vi "Item.vi"(8 "error in (no error)":errorcluster, 10 "Key":string, 11 "VariantAttribute in":refnum<class "MapImp.lvclass">) -> (0 "error out":errorcluster, 1 "Value":refnum<class>, 3 "VariantAttribute out":refnum<class "MapImp.lvclass">)   [LabVIEW 2013, in "LapDog.Collections.v1.Maps.lvlib" / "MapImp.lvclass"]
doc: "Returns a copy of the value associated with the given key.\n\nIf the key does not exist, error 510203 is returned."
uses:
  MapImp.lvclass
  MapImp.lvclass/MapImp.ctl
  LapDog.Collections.Common/LapDog.Collections.v1.Common.lvlib
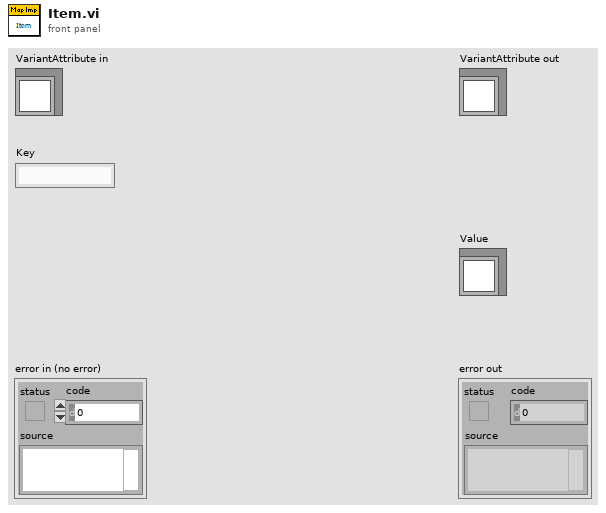
[diagram p1: front panel]
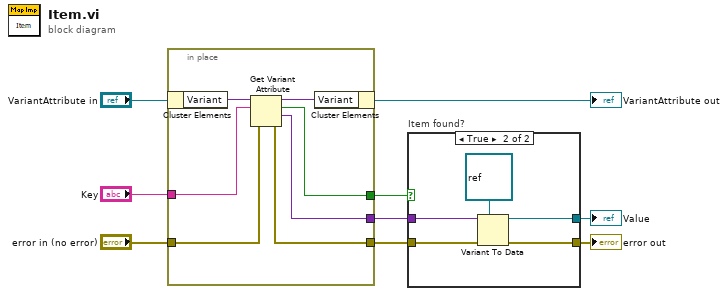
[diagram p0: block diagram]
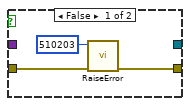
[diagram p2: hidden frame]
diagram:
  n1 = in-place {
    in-place-border: "error in (no error)" -> [w15]
    in-place-border: "Key" -> [w14]
    in-place-border: [w12] -> w4
    in-place-border: [w11] -> w3
    in-place-border: [w10] -> w1
    n2 = in-place-cluster #1("VariantAttribute in") -> ("Variant"=w16:variant)
    n3 = Get Variant Attribute(Variant=w16, name=w14, error in=w15) -> (duplicate Variant=w13:variant, found=w10:bool, value=w11:variant, error out=w12:errorcluster)  [unwired: 1 in]
    n4 = in-place-cluster #1("Variant"=w13) -> (→"VariantAttribute out":refnum<class "MapImp.lvclass">)
  }
  n5 = case "Item found?" shown="True" w1 {
    tunnel: [w18 w24] -> w5
    tunnel: w4 -> [w19 w23]
    tunnel: w3 -> [_ w22]
    tunnel: [_ w20] -> w2
    frame False {
      n6 = call "RaiseError.vi"("error in (no error)"=w19, "Error Code"=510203) -> ("error out"=w18:errorcluster)  [unwired: 9 in]
    }
    frame True {
      n7 = Variant To Data(error in=w23, type=refnum<class> refnum ("LabVIEW Object"), Variant=w22) -> (data=w20:refnum<class>, error out=w24:errorcluster)
    }
  }
  "error out" <- w5
  "Value" <- w2
